vi "FGV_Laser Power Calibration.vi"(7 "Input includes FOV sizes line? (T)":bool=TRUE, 8 "error in (no error)":errorcluster, 9 "Function":T1=enum."Read", 10 "Calibration Data in (% efficiency)":dbl[][](array[numeric])=[[-1.0, 148.1, 179.3, 262.9], [-0.8, 118.0, 140.7, 217.8], [-0.6, 90.0, 106.7, 183.1], [-0.4, 59.7, 68.6, 132.8], [-0.2, 27.9, 33.1, 74.0], [0.0, 0.0, 0.0, 0.0], [0.2, -32.0, -50.0, -50.2], [0.4, -65.7, -90.6, -118.9], [0.6, -98.2, -135.6, -196.7], [0.8, -131.7, -182.8, -291.7], [1.0, -168.7, -223.8, -376.0]]) -> (0 "error out":errorcluster, 1 "Real AOL Z":dbl[](array[numeric]), 2 "Calibration Data (% efficiency)":dbl[][](array[numeric]), 3 "Dwell time values (us)":dbl[](array[numeric]))   [LabVIEW 2013]
uses:
  Typedefs/Functional global standard states.ctl
  Typedefs/Read Write Enum.ctl
  Typedefs/Which path.ctl
  gl_Calibration globals.vi
  Program Files (x86)/National Instruments/LabVIEW 2013/user.lib/My Palettes.lib/Files & paths/Spreadsheet/Read From Spreadsheet File (DBL)-Mod.vi
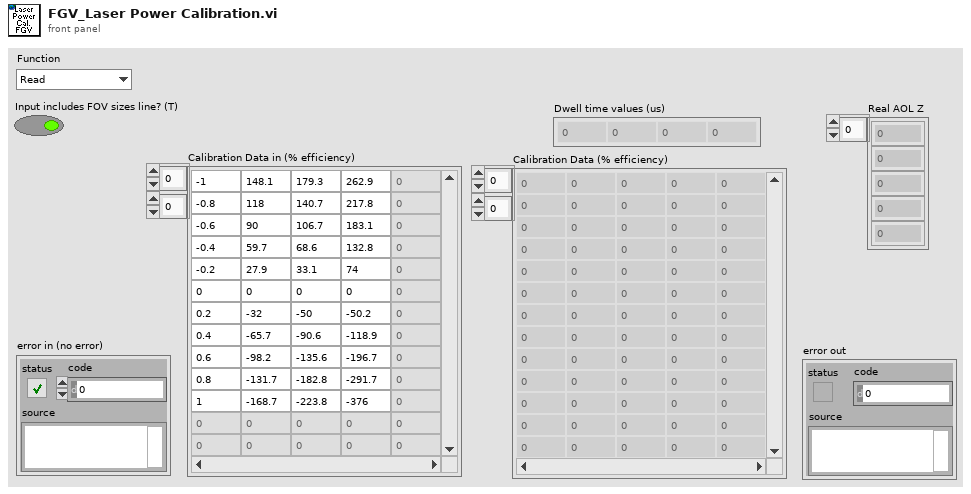
[diagram p1: front panel]
types:
  T1 = typedef "Functional global standard states.ctl" = enum16{"Initialise", "Read", "Write", "Load", "Save", "Clear"}
  T2 = typedef "Which path.ctl" = enum16{"Configuration Files", "Calibration Files", "Images", "Setup.ini", "Loaded User profile.ini", "User's-Previous session.ini", "New user profile.ini", "Selected User profile.ini", "User profiles folder", "Power meter scaling.txt", "FOV Cal.ini"}
  T3 = typedef "Read Write Enum.ctl" = enum16{"Read", "Write"}
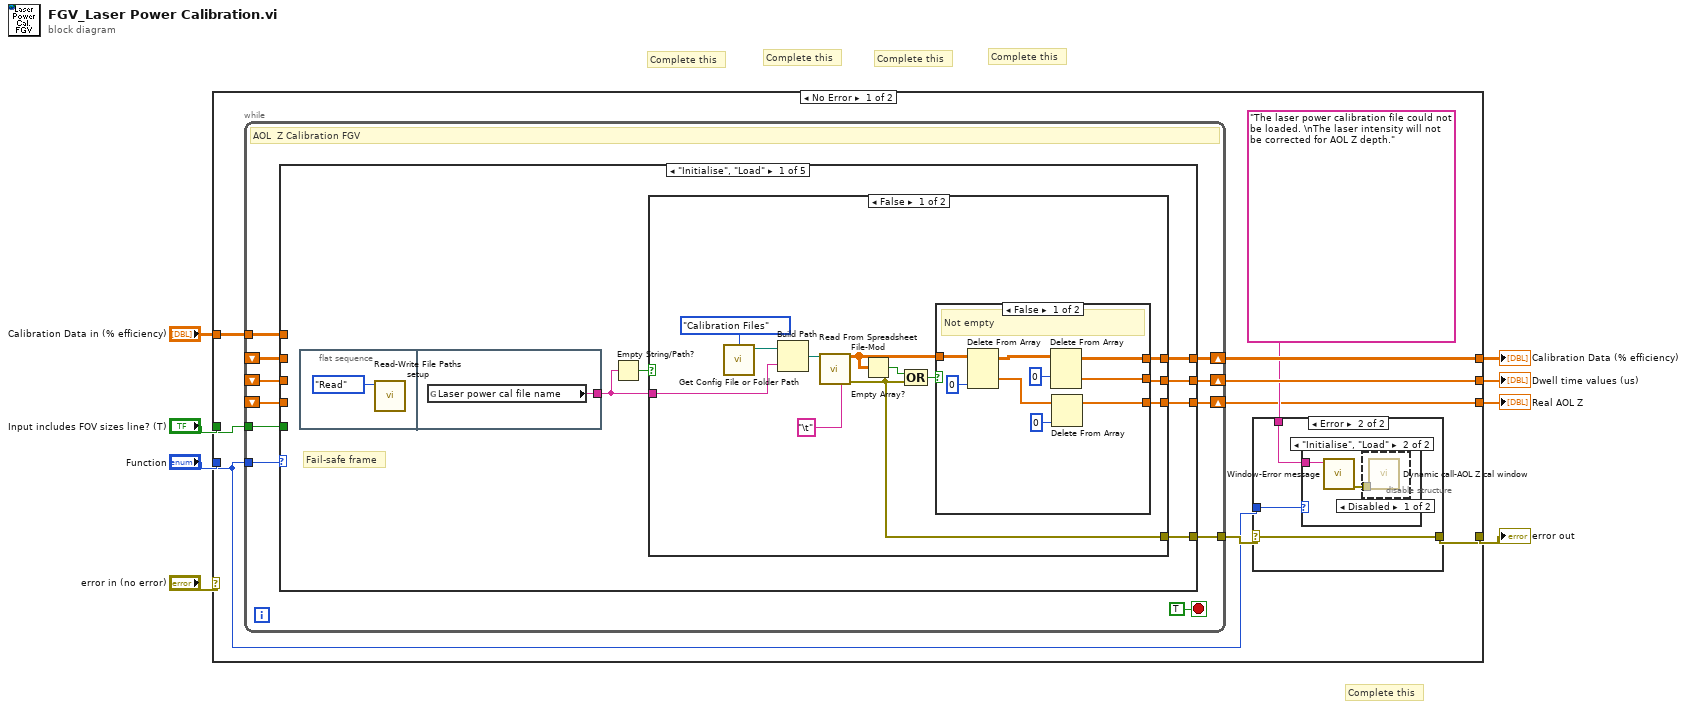
[diagram p0: block diagram]
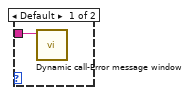
[diagram p3: hidden frame]
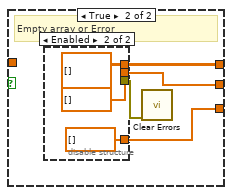
[diagram p5: hidden frame]
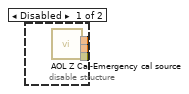
[diagram p6: hidden frame]
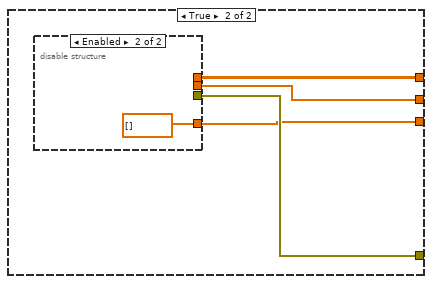
[diagram p7: hidden frame]
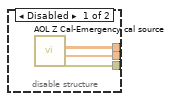
[diagram p8: hidden frame]
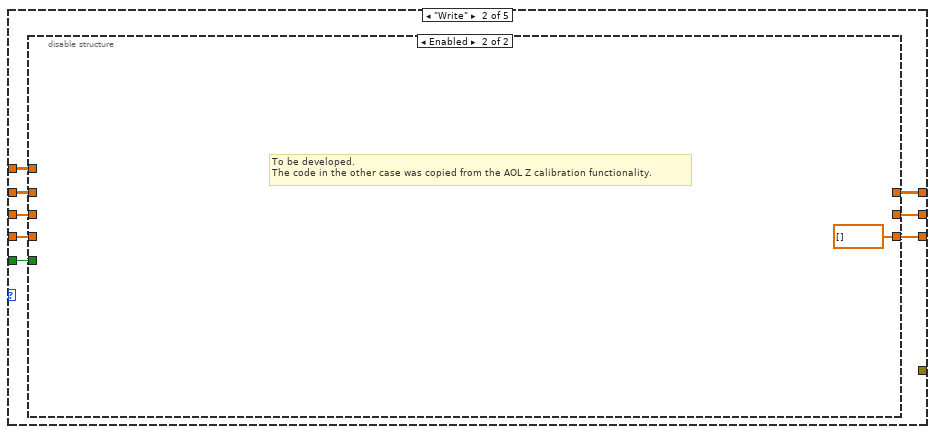
[diagram p9: hidden frame]
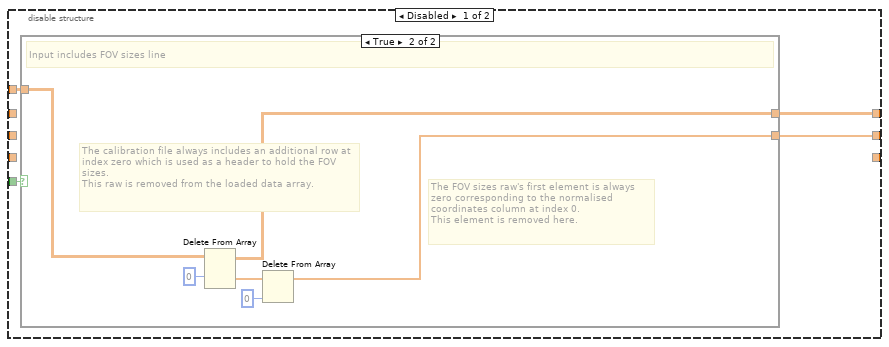
[diagram p10: hidden frame]
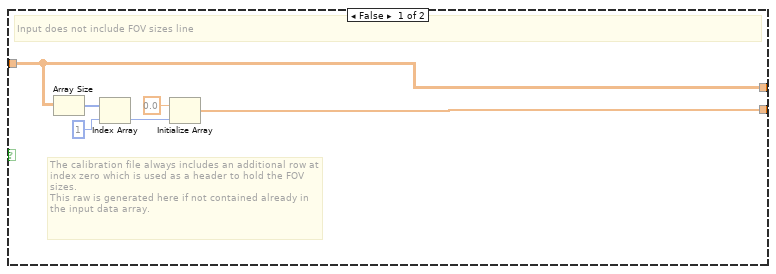
[diagram p11: hidden frame]
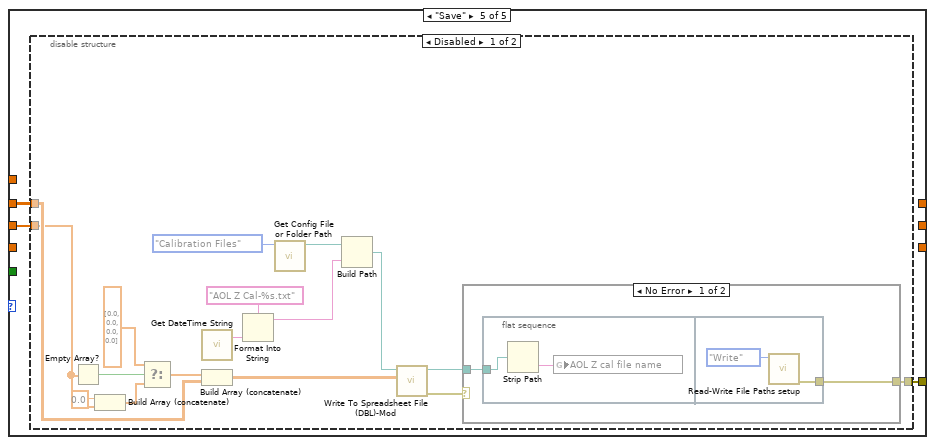
[diagram p14: hidden frame]
diagram:
  # "Complete this"
  # "Complete this"
  # "Complete this"
  # "Complete this"
  # "Complete this"
  n1 = case shown="No Error" "error in (no error)" {
    selector: "error in (no error)" -> [_ w142]
    tunnel: [w12 w142] -> w2
    tunnel: "Function" -> [w10 _]
    tunnel: "Calibration Data in (% efficiency)" -> [w17 _]
    tunnel: "Input includes FOV sizes line? (T)" -> [w16 _]
    tunnel: [w15 _] -> w5
    tunnel: [w14 _] -> w4
    tunnel: [w9 _] -> w1
    frame No Error {
      n2 = while {
        tunnel: w10 -> [w36]
        tunnel: w17 -> [w34]
        tunnel: w16 -> [w33]
        shift-right: [w32] -> w15
        shift-left: _ -> [w31]
        shift-right: [w30] -> w14
        shift-left: _ -> [w29]
        tunnel: [w28] -> w13
        shift-right: [w27] -> w9
        shift-left: _ -> [w26]
        stop <- TRUE stop-if-true
        # "AOL  Z Calibration FGV"
        n3 = case shown="\"Initialise\", \"Load\"" w36 {
          tunnel: [w38 _ _ _ w116] -> w28
          tunnel: w34 -> [_ w91 _ _ _]
          tunnel: w33 -> [_ w89 _ _ _]
          tunnel: [w42 w90 w109 w114 _] -> w32
          tunnel: w31 -> [_ w84 w109 w114 w117]
          tunnel: [w41 w88 w110 w113 _] -> w30
          tunnel: w29 -> [_ w85 w110 w113 w115]
          tunnel: [w37 w86 w111 w112 _] -> w27
          tunnel: w26 -> [_ w87 w111 w112 _]
          frame "Initialise", "Load" {
            # "Fail-safe frame"
            n4 = flat-sequence {
              tunnel: [w83] -> w40
              frame #0 {
                n5 = call "Read-Write File Paths setup.vi"("Function"=Read_Write_Enum."Read") -> ()  [unwired: 10 in, 1 out]
              }
              frame #1 {
                n6 = global read "gl_Calibration globals.vi" "Laser power cal file name"() -> (w83:string)
              }
            }
            n7 = Empty String/Path?(string/path=w40) -> (empty?=w39:bool)
            n8 = case shown="False" w39 {
              tunnel: [w52 w77] -> w42
              tunnel: [w51 w76] -> w41
              tunnel: w40 -> [w50 _]
              tunnel: [w46 w75] -> w38
              tunnel: [w43 w74] -> w37
              frame False {
                n9 = call "Get Config File or Folder Path.vi"("Which file or folder?"=Which_path."Calibration Files" ("Which path?")) -> ("File Path"=w53:path)  [unwired: 8 in, 2 out]
                n10 = Build Path(base path=w53, name or relative path=w50) -> (appended path=w49:path)
                n11 = call-poly "Read From Spreadsheet File-Mod.vi"("file path (dialog if empty)"=w49, "delimiter (\\t)"="\t" ("delimiter (\\t)")) -> ("all rows"=w45:dbl[][], "error out"=w46:errorcluster)  [unwired: 8 in, 4 out]
                n12 = Empty Array?(array=w45) -> (empty?=w48:bool)
                n13 = Compound Arithmetic op=OR(w48, w46) -> (w47:bool)
                n14 = case shown="False" w47 {
                  tunnel: w45 -> [w61 _]
                  tunnel: [w63 w67] -> w52
                  tunnel: [w55 w66] -> w51
                  tunnel: [w56 w64] -> w43
                  frame False {
                    # "Not empty"
                    n15 = Delete From Array(array=w61, index (col)=0 ("disabled index (col)")) -> (deleted portion=w59:dbl[], array with subset deleted=w60:dbl[][])  [unwired: 2 in]
                    n16 = Delete From Array(array=w60, index (row)=0) -> (deleted portion=w55:dbl[], array with subset deleted=w63:dbl[][])  [unwired: 2 in]
                    n17 = Delete From Array(array=w59, index=0) -> (array with subset deleted=w56:dbl[])  [unwired: 1 in, 1 out]
                  }
                  frame True {
                    # "Empty array or Error"
                    n18 = disable-structure shown="Enabled" {
                      disable-tunnel: [w70 dbl[][] [] ("Calibration Data")] -> w67
                      disable-tunnel: [w69 dbl[] [] ("FOV Sizes")] -> w66
                      disable-tunnel: [w68 _] -> w65
                      disable-tunnel: [_ dbl[] [] ("all rows")] -> w64
                      frame Disabled {
                        n19 = call "AOL Z Cal-Emergency cal source.vi"() -> ("error out"=w68:errorcluster, "FOV Sizes"=w69:dbl[], "Calibration Data"=w70:dbl[][])  [unwired: 9 in]
                      }
                      frame Enabled {
                      }
                    }
                    n20 = call <vilib>:"Clear Errors.vi"("error in (no error)"=w65) -> ()  [unwired: 6 in, 1 out]
                  }
                }
              }
              frame True {
                n21 = disable-structure shown="Enabled" {
                  disable-tunnel: [w80 _] -> w77
                  disable-tunnel: [w79 _] -> w76
                  disable-tunnel: [w78 _] -> w75
                  disable-tunnel: [_ dbl[] [] ("all rows")] -> w74
                  frame Disabled {
                    n22 = call "AOL Z Cal-Emergency cal source.vi"() -> ("error out"=w78:errorcluster, "FOV Sizes"=w79:dbl[], "Calibration Data"=w80:dbl[][])  [unwired: 9 in]
                  }
                  frame Enabled {
                  }
                }
              }
            }
          }
          frame "Write" {
            n23 = disable-structure shown="Enabled" {
              disable-tunnel: w91 -> [w95 _]
              disable-tunnel: [w94 _] -> w90
              disable-tunnel: w89 -> [w93 _]
              disable-tunnel: [w92 _] -> w88
              disable-tunnel: w87 -> [_ _]
              disable-tunnel: [_ dbl[] [] ("all rows")] -> w86
              disable-tunnel: w85 -> [_ _]
              disable-tunnel: w84 -> [_ _]
              frame Disabled {
                n24 = case shown="True" w93 {
                  tunnel: [w101 w102] -> w94
                  tunnel: w95 -> [w101 w103]
                  tunnel: [w96 w104] -> w92
                  frame False {
                    # "The calibration file always includes an additional row at index zero which is used as a header to hold the FOV sizes.\nThis raw is generated here if not contained already in the input data array."
                    # "Input does not include FOV sizes line"
                    n25 = Array Size(array=w101) -> (size(s)=w100:i32[])
                    n26 = Index Array(array=w100, index=1) -> (element=w98:i32)
                    n27 = Initialize Array(0.0 ("element"), w98) -> (w96:dbl[])
                  }
                  frame True {
                    # "The FOV sizes raw's first element is always zero corresponding to the normalised coordinates column at index 0.\nThis element is removed here."
                    # "The calibration file always includes an additional row at index zero which is used as a header to hold the FOV sizes.\nThis raw is removed from the loaded data array."
                    # "Input includes FOV sizes line"
                    n28 = Delete From Array(array=w103, index (row)=0) -> (deleted portion=w106:dbl[], array with subset deleted=w102:dbl[][])  [unwired: 2 in]
                    n29 = Delete From Array(array=w106, index=0) -> (array with subset deleted=w104:dbl[])  [unwired: 1 in, 1 out]
                  }
                }
              }
              frame Enabled {
                # "To be developed.\nThe code in the other case was copied from the AOL Z calibration functionality."
              }
            }
          }
          frame "Clear" {
          }
          frame "Read", Default {
          }
          frame "Save" {
            n30 = disable-structure shown="Disabled" {
              disable-tunnel: w117 -> [w126 _]
              disable-tunnel: [w125 _] -> w116
              disable-tunnel: w115 -> [w124 _]
              frame Disabled {
                n31 = Empty Array?(array=w124) -> (empty?=w129:bool)
                n32 = Build Array (concatenate)(0.0, w124) -> (w123:dbl[])
                n33 = Select(t=dbl[] [0.0, 0.0, 0.0, 0.0], s=w129, f=w123) -> (s? t:f=w127:dbl[])
                n34 = call "Get DateTime String.vi"() -> ("date/time string"=w133:string)  [unwired: 10 in, 1 out]
                n35 = Build Array (concatenate)(w127, w126) -> (w120:dbl[][])
                n36 = Format Into String(format string="AOL Z Cal-%s.txt", w133) -> (resulting string=w132:string)  [unwired: 2 in, 1 out]
                n37 = call "Get Config File or Folder Path.vi"("Which file or folder?"=Which_path."Calibration Files" ("Which path?")) -> ("File Path"=w130:path)  [unwired: 8 in, 2 out]
                n38 = Build Path(base path=w130, name or relative path=w132) -> (appended path=w121:path)
                n39 = call "Write To Spreadsheet File (DBL)-Mod.vi"("2D data"=w120, "file path (dialog if empty)"=w121) -> ("error out"=w119:errorcluster, "new file path (Not A Path if cancelled)"=w118:path)  [unwired: 8 in]
                n40 = case shown="No Error" w119 {
                  selector: w119 -> [_ w141]
                  tunnel: [w135 w141] -> w125
                  tunnel: w118 -> [w136 _]
                  frame No Error {
                    n41 = flat-sequence {
                      tunnel: w136 -> [w138]
                      tunnel: [w139] -> w135
                      frame #0 {
                        n42 = Strip Path(path=w138) -> (name=w137:string)  [unwired: 1 out]
                        n43 = global write "gl_Calibration globals.vi" "AOL Z cal file name"(w137) -> ()
                      }
                      frame #1 {
                        n44 = call "Read-Write File Paths setup.vi"("Function"=Read_Write_Enum."Write") -> ("error out"=w139:errorcluster)  [unwired: 10 in]
                      }
                    }
                  }
                  frame Error {
                  }
                }
              }
              frame Enabled {
                # "To be developed.\nThe code in the other case was copied from the AOL Z calibration functionality."
              }
            }
          }
        }
      }
      n45 = case shown="Error" w13 {
        selector: w13 -> [w18 w21]
        tunnel: [w18 w21] -> w12
        tunnel: "The laser power calibration file could not be loaded. \nThe laser intensity will not be corrected for AOL Z depth." ("Error Message") -> [_ w19]
        tunnel: w10 -> [_ w20]
        frame No Error {
        }
        frame Error {
          n46 = case shown="\"Initialise\", \"Load\"" w20 {
            tunnel: w19 -> [w22 w24]
            frame Default {
              n47 = call "Dynamic call-Error message window.vi"("Error Message"=w22) -> ()  [unwired: 10 in, 1 out]
            }
            frame "Initialise", "Load" {
              n48 = call "Window-Error message.vi"("Message"=w24) -> ("Error Out (no error)"=w23:errorcluster)  [unwired: 10 in]
              n49 = disable-structure shown="Disabled" {
                disable-tunnel: w23 -> [w25 _]
                frame Disabled {
                  n50 = call "Dynamic call-AOL Z cal window.vi"("error in (no error)"=w25) -> ()  [unwired: 10 in, 1 out]
                }
                frame Enabled {
                }
              }
            }
          }
        }
      }
    }
    frame Error {
    }
  }
  "error out" <- w2
  "Calibration Data (% efficiency)" <- w5
  "Dwell time values (us)" <- w4
  "Real AOL Z" <- w1
